vi "Get a Voltages.vi"(8 "error in":errorcluster, 9 "Selector":T1(ring), 11 "DMM Port":string) -> (0 "error out":errorcluster, 1 "Selected Measurement":dbl, 3 "Measurement Data":dbl[](array[numeric]))   [LabVIEW 2015]
uses:
  <instrlib>/Keithley 27XX/Keithley 27XX.lvlib
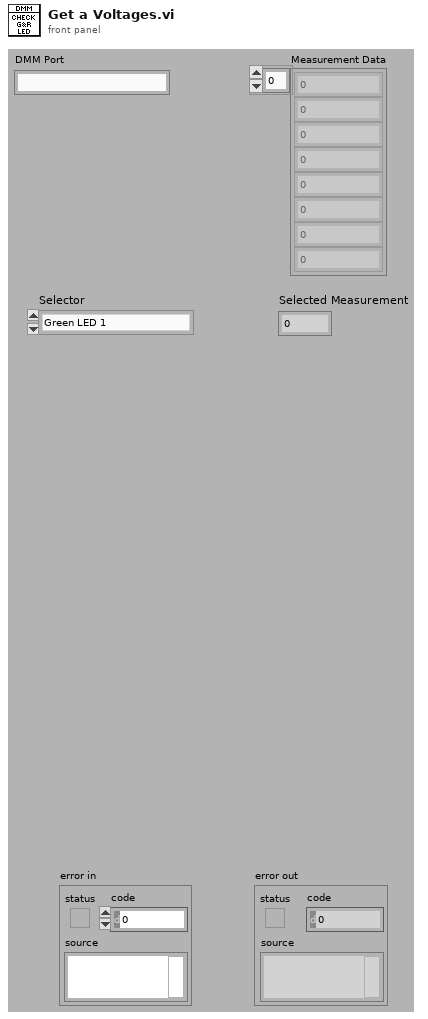
[diagram p1: front panel]
types:
  T1 = enum16{"Green LED 1", "Red LED", "VCELL", "VP2 TESTER", "TEMP TESTER", "Green LED 2"}
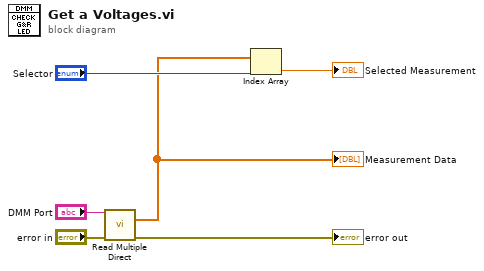
[diagram p0: block diagram]
diagram:
  n1 = call <instrlib>:"Read Multiple Direct.vi"("VISA resource name"="DMM Port", "error in (no error)"="error in") -> ("Measurement Data"=w1:dbl[], "error out"=→"error out":errorcluster)  [unwired: 8 in, 4 out]
  "Measurement Data" <- w1
  n2 = Index Array(array=w1, index="Selector") -> (element=→"Selected Measurement":dbl)
